vi "Wait Until Text In.vi"(1 "command text in":string[](array[string])) -> (0 "Wait Until Ctr":T1={"Available Data"=[], "Target Value"=0.0, "Condition"=enum."= target value", "xxx%"=0.0, "Timeout (sec)"=30000.0, "selected index"=0, "initial wait (sec)"=0.0})   [LabVIEW 2025]
doc: "Author: Scott Hannahs <sth@magnet.fsu.edu>\n\nThis software is licensed for use under the “MIT License\"\nCopyright (c) 2025 Scott Hannahs, sth@sth@magnet.sthnet.net\n\nPermission is hereby granted, free of charge, to any person obtaining a copy of this software and associated documentation files (the \"Software\"), to deal in the Software without restriction, including without limitation the rights to use, copy, modify, merge, publish, distribute, sublicense, and/or sell copies of the Software, and to permit persons to whom the Software is furnished to do so, subject to the following conditions: The above copyright notice and this permission notice shall be included in all copies or substantial portions of the Software.\n\nTHE SOFTWARE IS PROVIDED \"AS IS\", WITHOUT WARRANTY OF ANY KIND, EXPRESS OR IMPLIED, INCLUDING BUT NOT LIMITED TO THE WARRANTIES OF MERCHANTABILITY, FITNESS FOR A PARTICULAR PURPOSE AND NONINFRINGEMENT. IN NO EVENT SHALL THE AUTHORS OR COPYRIGHT HOLDERS BE LIABLE FOR ANY CLAIM, DAMAGES OR OTHER LIABILITY, WHETHER IN AN ACTION OF CONTRACT, TORT OR OTHERWISE, ARISING FROM, OUT OF OR IN CONNECTION WITH THE SOFTWARE OR THE USE OR OTHER DEALINGS IN THE SOFTWARE."
uses:
  Wait Until.ctl
  Wait Until condition.ctl
panel:
  # "Wait Until Command"
  # "This command waits until 'DATA' value in NML Data Acquisition program meets user specified the condition."
  # "Select DATA to monitor"
  # "Enter Target value"
  # "Specifiy 'wait until' condition"
  # "Wait until DATA  is"
  # "(Specify"
  # "if necessary)"
  # "Enter 'Time out' here"
  # "sec"
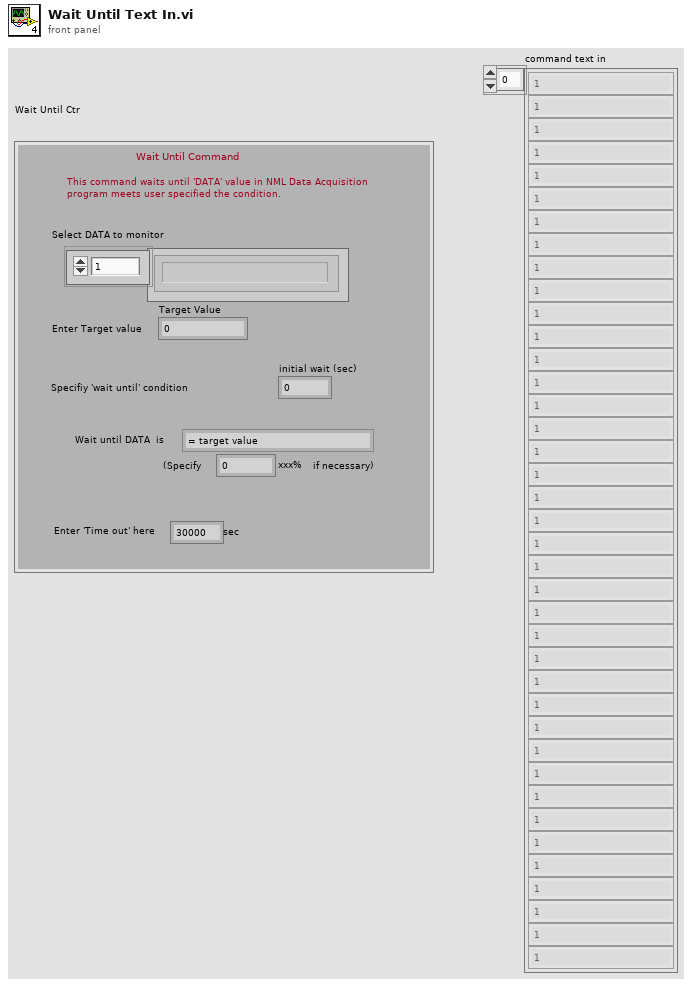
[diagram p1: front panel]
types:
  T1 = typedef "Wait Until.ctl" = cluster{"Available Data":string[], "Target Value":dbl, "Condition":T2, "xxx%":dbl, "Timeout (sec)":dbl, "selected index":u32, "initial wait (sec)":dbl}
  T2 = typedef "Wait Until condition.ctl" = enum16{"within xxx% of target value", "<= target value", ">= target value", "= target value"}
  T3 = cluster{"command text in[0]":string, "command text in[1]":string, "command text in[2]":string, "command text in[3]":string, "command text in[4]":string, "command text in[5]":string, "command text in[6]":string, "command text in[7]":string, "command text in[8]":string, "command text in[9]":string, "command text in[10]":string, "command text in[11]":string, "command text in[12]":string, "command text in[13]":string, "command text in[14]":string, "command text in[15]":string, "command text in[16]":string, "command text in[17]":string, "command text in[18]":string, "command text in[19]":string, "command text in[20]":string, "command text in[21]":string, "command text in[22]":string, "command text in[23]":string, "command text in[24]":string, "command text in[25]":string}
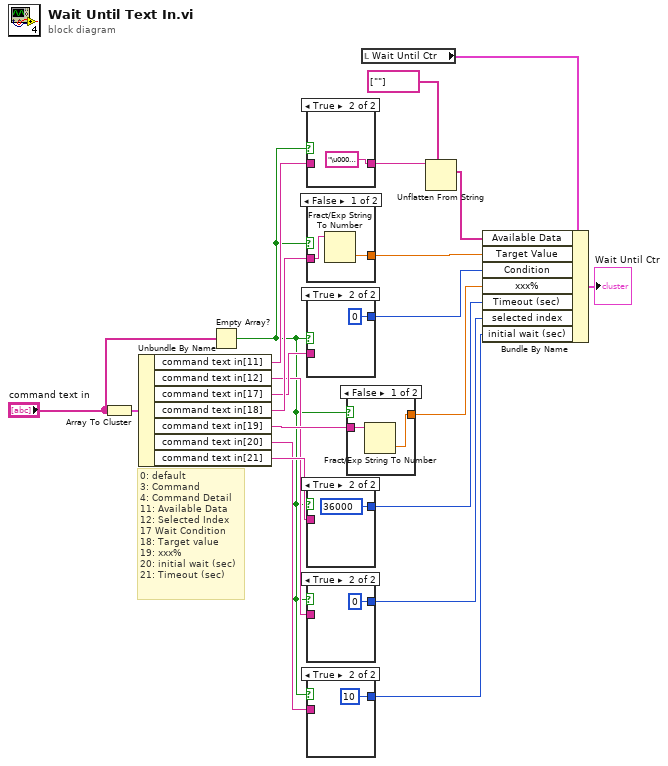
[diagram p0: block diagram]
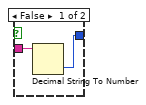
[diagram p2: hidden frame]
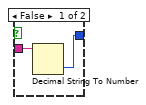
[diagram p4: hidden frame]
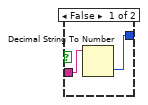
[diagram p5: hidden frame]
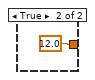
[diagram p6: hidden frame]
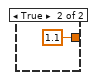
[diagram p7: hidden frame]
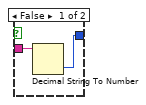
[diagram p8: hidden frame]
diagram:
  # "0: default\n3: Command\n4: Command Detail\n11: Available Data\n12: Selected Index\n17 Wait Condition\n18: Target value\n19: xxx%\n20: initial wait (sec)\n21: Timeout (sec)"
  n1 = Array To Cluster(array="command text in") -> (cluster=w21:T3)
  n2 = Unbundle By Name(w21) -> ("command text in[11]"=w4:string, "command text in[12]"=w9:string, "command text in[17]"=w10:string, "command text in[18]"=w12:string, "command text in[19]"=w14:string, "command text in[20]"=w3:string, "command text in[21]"=w19:string)
  n3 = Empty Array?(array="command text in") -> (empty?=w2:bool)
  n4 = case shown="True" w2 {
    tunnel: [w22 "\u0000\u0000\u0000\u0001\u0000\u0000\u0000\u00011" ("binary string")] -> w6
    tunnel: w4 -> [w22 _]
    frame False {
    }
    frame True {
    }
  }
  n5 = case shown="False" w2 {
    tunnel: w12 -> [w25 _]
    tunnel: [w24 12.0] -> w13
    frame False {
      n6 = Fract/Exp String To Number(string=w25) -> (number=w24:dbl)  [unwired: 3 in, 1 out]
    }
    frame True {
    }
  }
  n7 = case shown="True" w2 {
    tunnel: w10 -> [w28 _]
    tunnel: [w27 0] -> w11
    frame False {
      n8 = Decimal String To Number(string=w28) -> (number=w27:i32)  [unwired: 2 in, 1 out]
    }
    frame True {
    }
  }
  n9 = case shown="True" w2 {
    tunnel: [w30 36000] -> w16
    tunnel: w19 -> [w31 _]
    frame False {
      n10 = Decimal String To Number(string=w31) -> (number=w30:i32)  [unwired: 2 in, 1 out]
    }
    frame True {
    }
  }
  n11 = case shown="True" w2 {
    tunnel: w9 -> [w34 _]
    tunnel: [w33 0] -> w8
    frame False {
      n12 = Decimal String To Number(string=w34) -> (number=w33:i32)  [unwired: 2 in, 1 out]
    }
    frame True {
    }
  }
  n13 = case shown="True" w2 {
    tunnel: [w36 10] -> w1
    tunnel: w3 -> [w37 _]
    frame False {
      n14 = Decimal String To Number(string=w37) -> (number=w36:i32)  [unwired: 2 in, 1 out]
    }
    frame True {
    }
  }
  n15 = case shown="False" w2 {
    tunnel: w14 -> [w40 _]
    tunnel: [w39 1.1] -> w15
    frame False {
      n16 = Fract/Exp String To Number(string=w40) -> (number=w39:dbl)  [unwired: 3 in, 1 out]
    }
    frame True {
    }
  }
  n17 = local read "Wait Until Ctr"() -> (w18:T1)
  n18 = Unflatten From String(type=string[] [""] ("Control"), binary string=w6) -> (value=w5:string[])  [unwired: 3 in, 2 out]
  n19 = Bundle By Name(cluster=w18, "Available Data"=w5, "Target Value"=w13, "Condition"=w11, "xxx%"=w15, "Timeout (sec)"=w16, "selected index"=w8, "initial wait (sec)"=w1) -> (→"Wait Until Ctr":T1)
